vi "Bundle.vi"(8 "error in (no error)":errorcluster, 10 "Message":refnum<class "Message.lvclass">, 11 "Targetted Msg in":refnum<class "Sender Msg.lvclass">) -> (0 "error out":errorcluster, 3 "Targetted Msg out":refnum<class "Sender Msg.lvclass">)   [LabVIEW 2020, in "Publisher.lvlib" / "Sender Msg.lvclass"]
doc: "Configure 'Addressed Msg' for execution."
uses:
  Sender Msg.lvclass
  PPL/HDH.Actor Framework.Core.Actor.lvlibp/1abvi3w/vi.lib/ActorFramework/Message/Message.lvclass
  Sender Msg.lvclass/Sender Msg.ctl
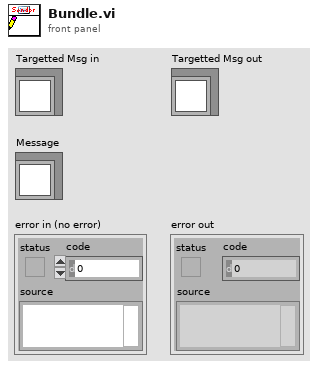
[diagram p1: front panel]
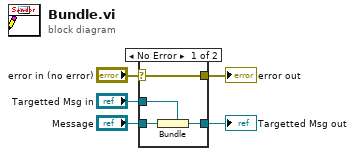
[diagram p0: block diagram]
diagram:
  n1 = case shown="No Error" "error in (no error)" {
    selector: "error in (no error)" -> [w9 w10]
    tunnel: [w9 w10] -> w4
    tunnel: [w7 w11] -> w2
    tunnel: "Targetted Msg in" -> [w8 w11]
    tunnel: "Message" -> [w6 _]
    frame No Error {
      n2 = Bundle(cluster=w8, w6) -> (w7:refnum<class "Sender Msg.lvclass">)
    }
    frame Error {
    }
  }
  "error out" <- w4
  "Targetted Msg out" <- w2
